vi "num2stringcentsSubVI.vi"(11 "Num":dbl) -> (3 "String with cents":string)   [LabVIEW 2019]
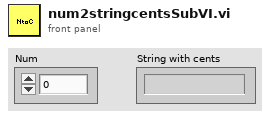
[diagram p1: front panel]
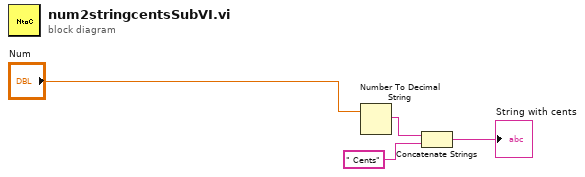
[diagram p0: block diagram]
diagram:
  n1 = Number To Decimal String(number="Num") -> (decimal integer string=w2:string)  [unwired: 1 in]
  n2 = Concatenate Strings(w2, " Cents" ("string")) -> (→"String with cents":string)
